vi "Post-Install Custom Action.vi"(10 "Variant":variant) -> (0 "error out":errorcluster)   [LabVIEW 2014]
uses:
  directory type.ctl
  <vilib>/regexp/Match Regular Expression.xnode
  <vilib>/zip/NI_Unzip.lvlib
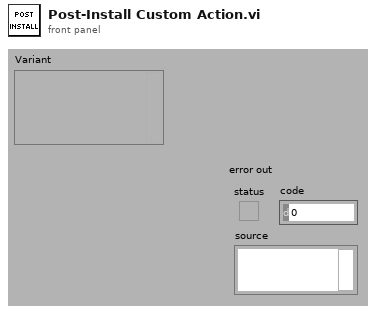
[diagram p1: front panel]
types:
  T1 = typedef "directory type.ctl" = i32
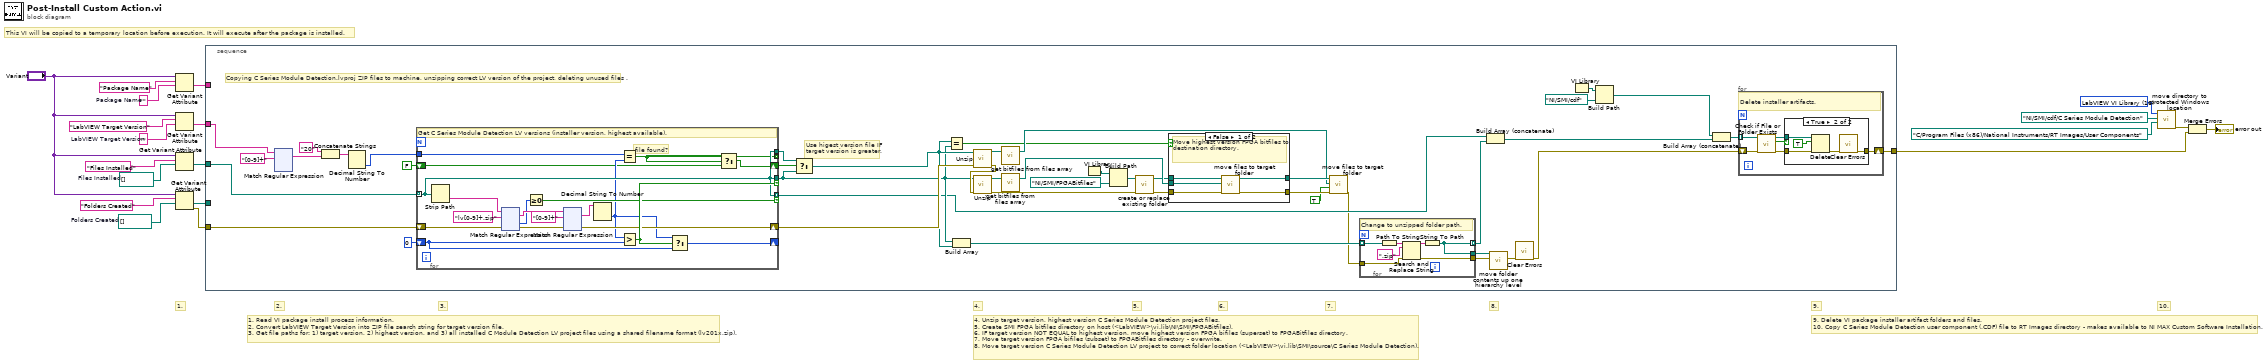
[diagram p0: block diagram]
diagram:
  w3 = path[] []  # Folders Created
  w4 = path[] []  # Files Installed
  w9 = T1 16 items=["User Home", "User Desktop", "User Documents", "User Application Data", "User Preferences", "User Temporary", "Public Documents", "Public Application Data", "Public Preferences", "System Core Libraries", "System Installed Libraries", "Application Files", "Boot Volume Root", "Public Cache", "LabVIEW Default Directory", "LabVIEW Default Data", "LabVIEW VI Library", "Application Directory"] ("system directory (<LabVIEW>/vi.lib)")
  w18 = ""  # LabVIEW Target Version
  w19 = ""  # Package Name
  # "9. Delete VI package installer artifact folders and files.\n10. Copy C Series Module Detection user component (.CDF) file to RT Images directory - makes available to NI MAX Custom Software Installation."
  # "8."
  # "7."
  # "6."
  # "5."
  # "9."
  # "10."
  # "4. Unzip target version, highest version C Series Module Detection project files.\n5. Create SMI FPGA bitfiles directory on host (<LabVIEW>\\vi.lib\\NI\\SMI\\FPGABitfiles).\n6. IF target version NOT EQUAL to highest version, move highest version FPGA bifiles (superset) to FPGABitfiles directory.\n7. Move target version FPGA bifiles (subset) to FPGABitfiles directory - overwrite.\n8. Move target version C Series Module Detection LV project to correct folder location (<LabVIEW>\\vi.lib\\SMI\\source\\C Series Module Detection)."
  # "4."
  # "3."
  # "2."
  # "1."
  # "1. Read VI package install process information.\n2. Convert LabVIEW Target Version into ZIP file search string for target version file.\n3. Get file paths for: 1) target version, 2) highest version, and 3) all installed C Module Detection LV project files using a shared filename format (lv201x.zip)."
  # "This VI will be copied to a temporary location before execution. It will execute after the package is installed."
  n1 = Get Variant Attribute(Variant="Variant", name="Package Name", default value (empty Variant)=w19) -> (value=w17:string)  [unwired: 1 in, 3 out]
  n2 = Get Variant Attribute(Variant="Variant", name="LabVIEW Target Version", default value (empty Variant)=w18) -> (value=w16:string)  [unwired: 1 in, 3 out]
  n3 = Get Variant Attribute(Variant="Variant", name="Files Installed", default value (empty Variant)=w4) -> (value=w14:path[])  [unwired: 1 in, 3 out]
  n4 = Get Variant Attribute(Variant="Variant", name="Folders Created", default value (empty Variant)=w3) -> (value=w15:path[], error out=w5:errorcluster)  [unwired: 1 in, 2 out]
  n5 = stacked-sequence {
    tunnel: w17 -> [_]
    tunnel: w16 -> [w62]
    tunnel: w14 -> [w64]
    tunnel: w15 -> [_]
    tunnel: [w61] -> w6
    tunnel: w5 -> [w63]
    frame #0 {
      # "Use higest version file IF\ntarget version is greater."
      # "Copying C Series Module Detection.lvproj ZIP files to machine, unzipping correct LV version of the project, deleting unused files ."
      n6 = xnode "Match Regular Expression"("input string"=w62, "regular expression"="[0-9]+") -> ("whole match"=w28:string)  [unwired: 4 in, 4 out]
      n7 = Concatenate Strings("20", w28) -> (w25:string)
      n8 = Decimal String To Number(string=w25) -> (number=w24:i32)  [unwired: 2 in, 1 out]
      n9 = for {
        tunnel: w64 -> [w185] mode=indexing
        shift-right: [w193] -> _
        shift-left: 0 -> [w192]
        tunnel: [w185] -> w43 if=w191
        shift-right: [w188] -> w60
        shift-left: w63 -> [w190]
        tunnel: [w185] -> w21 if=w180
        tunnel: [w185] -> w42 mode=indexing if=w184
        tunnel: w24 -> [w183]
        tunnel: [w180] -> _ mode=indexing
        shift-right: [w181] -> w22
        shift-left: FALSE -> [w179]
        # "file found?"
        # "Get C Series Module Detection LV versions (installer version, highest available)."
        n10 = Strip Path(path=w185) -> (name=w196:string)  [unwired: 1 out]
        n11 = xnode "Match Regular Expression"("input string"=w196, "regular expression"="lv[0-9]+.zip", "error in"=w190) -> ("whole match"=w187:string, "offset past match"=w186:i32, "error out"=w189:errorcluster)  [unwired: 3 in, 2 out]
        n12 = Greater Or Equal To 0?(x=w186) -> (x >= 0?=w184:bool)
        n13 = xnode "Match Regular Expression"("input string"=w187, "regular expression"="[0-9]+", "error in"=w189) -> ("whole match"=w194:string, "error out"=w188:errorcluster)  [unwired: 3 in, 3 out]
        n14 = Decimal String To Number(string=w194) -> (number=w182:i32)  [unwired: 2 in, 1 out]
        n15 = Equal?(x=w183, y=w182) -> (x = y?=w180:bool)
        n16 = Greater?(x=w182, y=w192) -> (0:w191:bool)
        n17 = Select(t=w182, s=w191, f=w192) -> (s? t:f=w193:i32)
        n18 = Select(t=w180, s=w180, f=w179) -> (s? t:f=w181:bool)
      }
      n19 = Select(t=w21, s=w22, f=w43) -> (s? t:f=w44:path)
      n20 = Equal?(x=w44, y=w43) -> (x = y?=w45:bool)
      n21 = Build Array(w43, w44) -> (w41:path[])
      n22 = call <vilib>:"Unzip.vi"("error in (no error)"=w60, "Zip file"=w44) -> ("error out"=w59:errorcluster, "Unzipped files"=w56:path[])  [unwired: 7 in, 1 out]
      n23 = call <vilib>:"Unzip.vi"("error in (no error)"=w59, "Zip file"=w43) -> ("error out"=w48:errorcluster, "Unzipped files"=w55:path[])  [unwired: 7 in, 1 out]
      n24 = call "get bitfiles from files array.vi"("file paths"=w56) -> ("FPGA bitfiles"=w51:path[])  [unwired: 2 in]
      n25 = call "get bitfiles from files array.vi"("file paths"=w55) -> ("FPGA bitfiles"=w54:path[])  [unwired: 2 in]
      n26 = VI Library() -> (path=w57:path)
      n27 = Build Path(base path=w57, name or relative path=path "NI/SMI/FPGABitfiles" ("directory name (relative to system directory)")) -> (appended path=w49:path)
      n28 = call "create or replace existing folder.vi"("error in"=w48, "path"=w49) -> ("error out"=w46:errorcluster, "created path"=w47:path)  [unwired: 8 in]
      n29 = case shown="False" w45 {
        tunnel: w54 -> [w437 _]
        tunnel: [w436 w439] -> w53
        tunnel: [w435 w438] -> w52
        tunnel: w47 -> [w434 w439]
        tunnel: w46 -> [w433 w438]
        frame False {
          # "Move highest version FPGA bitfiles to destination directory."
          n30 = call "move files to target folder.vi"("error in"=w433, "files"=w437, "target folder"=w434) -> ("error out"=w435:errorcluster, "target folder duplicate"=w436:path)  [unwired: 6 in, 1 out]
        }
        frame True {
        }
      }
      n31 = call "move files to target folder.vi"("error in"=w52, "overwrite (F)"=TRUE, "files"=w51, "target folder"=w53) -> ("error out"=w38:errorcluster)  [unwired: 5 in, 2 out]
      n32 = for {
        tunnel: w41 -> [w429] mode=indexing
        tunnel: [w428] -> w37 mode=indexing
        tunnel: [w428] -> w40
        tunnel: w38 -> [w427]
        tunnel: [w426] -> w39
        # "Change to unzipped folder path."
        n33 = Path To String(path=w429) -> (string=w432:string)
        n34 = Search and Replace String(input string=w432, search string=".zip", error in=w427) -> (result string=w430:string, error out=w426:errorcluster)  [unwired: 5 in, 2 out]
        n35 = String To Path(string=w430) -> (path=w428:path)
      }
      n36 = Build Array (concatenate)(w42, w37) -> (w31:path[])
      n37 = call "move folder contents up one hierarchy level.vi"("error in"=w39, "file"=w40) -> ("error out"=w34:errorcluster)  [unwired: 9 in]
      n38 = call <vilib>:"Clear Errors.vi"("error in (no error)"=w34) -> ("error out"=w33:errorcluster)  [unwired: 5 in, 1 out]
      n39 = VI Library() -> (path=w36:path)
      n40 = Build Path(base path=w36, name or relative path=path "NI/SMI/cdf") -> (appended path=w32:path)
      n41 = Build Array (concatenate)(w32, w31) -> (w30:path[])
      n42 = for {
        tunnel: w30 -> [w441] mode=indexing
        shift-right: [w440] -> w61
        shift-left: w33 -> [w442]
        # "Delete installer artifacts."
        n43 = call <vilib>:"Check if File or Folder Exists.vi"("error in (no error)"=w442, "path"=w441) -> ("error out"=w444:errorcluster, "file or folder exists?"=w445:bool, "dup path"=w443:path)  [unwired: 7 in]
        n44 = case shown="True" w445 {
          tunnel: [w446 w449] -> w440
          tunnel: w443 -> [_ w448]
          tunnel: w444 -> [w446 w447]
          frame False {
          }
          frame True {
            n45 = Delete(path (use dialog)=w448, entire hierarchy (F)=TRUE, error in=w447) -> (error out=w450:errorcluster)  [unwired: 2 in, 2 out]
            n46 = call <vilib>:"Clear Errors.vi"("error in (no error)"=w450) -> ("error out"=w449:errorcluster)  [unwired: 5 in, 1 out]
          }
        }
      }
    }
  }
  n47 = call "move directory to protected Windows location.vi"("Destination directory"=path "C:/Program Files (x86)/National Instruments/RT Images/User Components", "directory name (relative to system directory)"=path "NI/SMI/cdf/C Series Module Detection", "system directory (<LabVIEW>/vi.lib)"=w9) -> ("error out"=w10:errorcluster)  [unwired: 6 in, 2 out]
  n48 = Merge Errors(w10, w6) -> (→"error out":errorcluster)
